vi "Initialise.vi"(8 "error in (no error)":errorcluster, 11 "Actor in":refnum<class "Info View.lvclass">) -> (0 "error out":errorcluster, 3 "Actor out":refnum<class "Info View.lvclass">, 5 "Observers":cluster{"Actor":refnum<event-registration>})   [LabVIEW 2015, in "Info View.lvclass"]
uses:
  Info View.lvclass
  Re-use Libraries/Minimal Actor Framework/Messaging/Message/Message.lvclass
  Re-use Libraries/Utility/Utility.lvlib
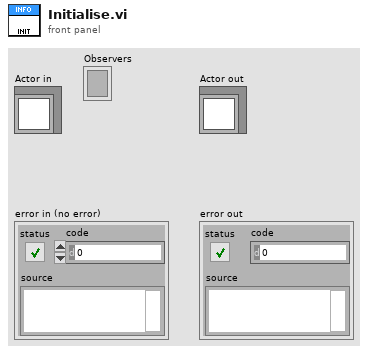
[diagram p1: front panel]
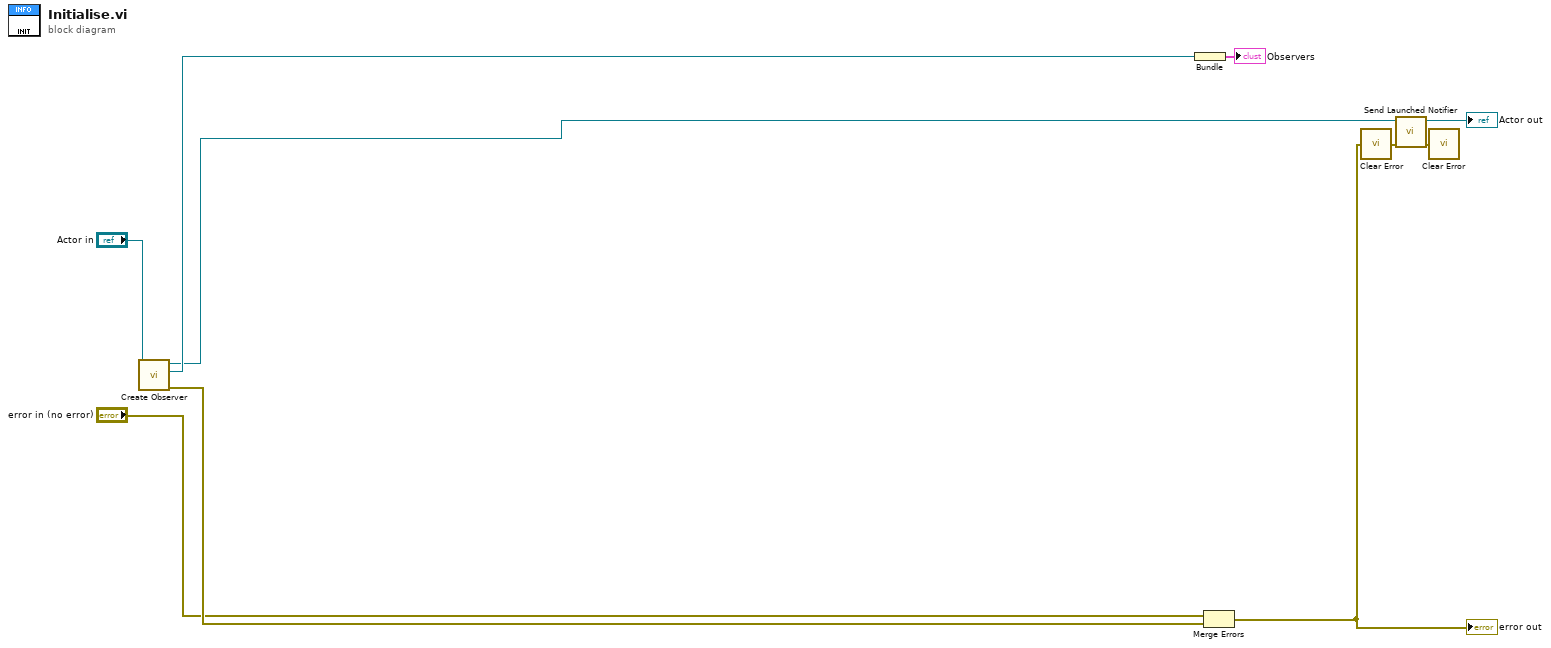
[diagram p0: block diagram]
diagram:
  n1 = call-dynamic "Create Observer.vi"("Actor in"="Actor in") -> ("error out"=w8:errorcluster, "Actor"=w3:refnum<event-registration>, "Actor out"=w1:refnum<class "Info View.lvclass">)  [unwired: 8 in]
  n2 = Bundle("Actor"=w3) -> (→"Observers":cluster{"Actor":refnum<event-registration>})  [unwired: 1 in]
  n3 = Merge Errors("error in (no error)", w8) -> (w7:errorcluster)
  "error out" <- w7
  n4 = call "Clear Error.vi"("error in (no error)"=w7) -> ("error out"=w6:errorcluster)
  n5 = call-dynamic "Send Launched Notifier.vi"("error in (no error)"=w6, "Actor in"=w1) -> ("error out"=w5:errorcluster, "Actor out"=→"Actor out":refnum<class "Info View.lvclass">)  [unwired: 8 in]
  n6 = call "Clear Error.vi"("error in (no error)"=w5) -> ()  [unwired: 1 out]
